vi "hmi_cheesy_drive.vi"(9 "Quick Turn":bool, 10 "Wheel":dbl, 11 "Throttle":dbl) -> (3 "Drive Data":cluster{"Left":dbl, "Right":dbl})   [LabVIEW 2011]
panel:
  in  "Speedturn_Sens_High":dbl=0.6
  in  "Speedturn_Sens_High max":dbl=0.6
  in  "Speedturn_Sens_Low max":dbl=0.6
  in  "gear shift state":enum16{"low", "high"}(ring)
  in  "Quickturn_Sens_High":dbl=1.0
  in  "Speedturn_Sens_Low":dbl=0.6
  in  "Quickturn_Sens_Low":dbl=1.0
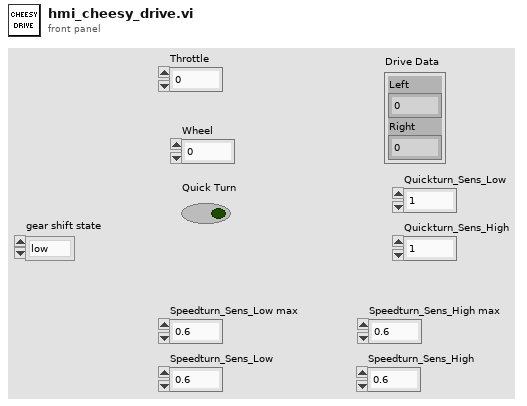
[diagram p1: front panel]
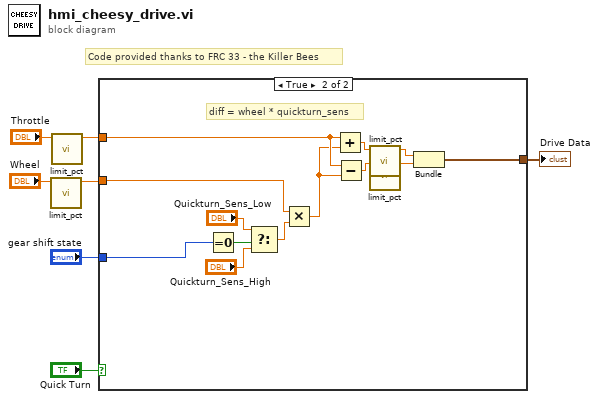
[diagram p0: block diagram]
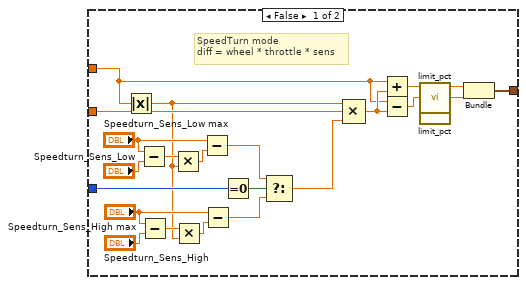
[diagram p2: hidden frame]
diagram:
  # "Code provided thanks to FRC 33 - the Killer Bees"
  n1 = call "limit_pct.vi"("PCT"="Wheel") -> ("PCT Out"=w3:dbl)  [unwired: 10 in]
  n2 = call "limit_pct.vi"("PCT"="Throttle") -> ("PCT Out"=w5:dbl)  [unwired: 10 in]
  n3 = case shown="True" "Quick Turn" {
    tunnel: w3 -> [w28 w38]
    tunnel: w5 -> [w11 w37]
    tunnel: [w26 w35] -> w7
    tunnel: "gear shift state" -> [w21 w30]
    frame False {
      # "SpeedTurn mode\ndiff = wheel * throttle * sens"
      n4 = Absolute Value(x=w11) -> (abs(x)=w8:dbl)
      n5 = Subtract(x="Speedturn_Sens_Low max", y="Speedturn_Sens_Low") -> (x-y=w18:dbl)
      n6 = Subtract(x="Speedturn_Sens_High max", y="Speedturn_Sens_High") -> (x-y=w13:dbl)
      n7 = Multiply(x=w18, y=w8) -> (x*y=w16:dbl)
      n8 = Multiply(x=w13, y=w8) -> (x*y=w15:dbl)
      n9 = Subtract(x="Speedturn_Sens_Low max", y=w16) -> (x-y=w9:dbl)
      n10 = Subtract(x="Speedturn_Sens_High max", y=w15) -> (x-y=w10:dbl)
      n11 = Equal To 0?(x=w21) -> (x = 0?=w29:bool)
      n12 = Select(t=w9, s=w29, f=w10) -> (s? t:f=w20:dbl)
      n13 = Compound Arithmetic op=MULTIPLY(w8, w28, w20) -> (w27:dbl)
      n14 = Add(x=w11, y=w27) -> (x+y=w24:dbl)
      n15 = Subtract(x=w11, y=w27) -> (x-y=w23:dbl)
      n16 = call "limit_pct.vi"("PCT"=w24) -> ("PCT Out"=w25:dbl)  [unwired: 10 in]
      n17 = call "limit_pct.vi"("PCT"=w23) -> ("PCT Out"=w22:dbl)  [unwired: 10 in]
      n18 = Bundle("PCT Out"=w25, "PCT Out"=w22) -> (w26:cluster{"PCT Out":dbl, "PCT Out":dbl})  [unwired: 1 in]
    }
    frame True {
      # "diff = wheel * quickturn_sens"
      n19 = Equal To 0?(x=w30) -> (x = 0?=w40:bool)
      n20 = Select(t="Quickturn_Sens_Low", s=w40, f="Quickturn_Sens_High") -> (s? t:f=w39:dbl)
      n21 = Multiply(x=w38, y=w39) -> (x*y=w36:dbl)
      n22 = Add(x=w37, y=w36) -> (x+y=w33:dbl)
      n23 = Subtract(x=w37, y=w36) -> (x-y=w31:dbl)
      n24 = call "limit_pct.vi"("PCT"=w33) -> ("PCT Out"=w34:dbl)  [unwired: 10 in]
      n25 = call "limit_pct.vi"("PCT"=w31) -> ("PCT Out"=w32:dbl)  [unwired: 10 in]
      n26 = Bundle("PCT Out"=w34, "PCT Out"=w32) -> (w35:cluster{"PCT Out":dbl, "PCT Out":dbl})  [unwired: 1 in]
    }
  }
  "Drive Data" <- w7
